vi "Get Column Config.vi"(8 "error in (no error)":errorcluster, 11 "Table Configuration Interface in":refnum<class "Table Configuration Interface.lvclass">) -> (0 "error out":errorcluster, 2 "Column Configuration":refnum<class "Column Configuration.lvclass">, 3 "Table Configuration Interface out":refnum<class "Table Configuration Interface.lvclass">)   [LabVIEW 2020, in "Table.lvlib" / "Table Configuration Interface.lvclass"]
uses:
  Table Configuration Interface.lvclass
  Column Libraries/Basic Columns/Column Configuration/Basic Column Configuration Class/Column Configuration.lvclass
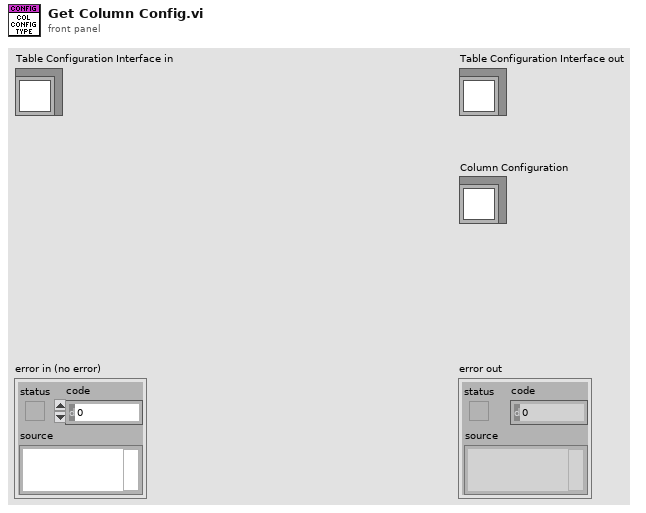
[diagram p1: front panel]
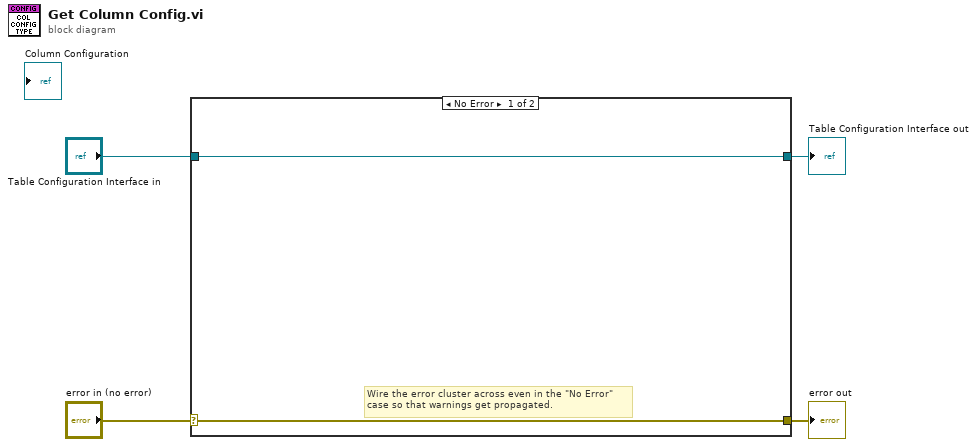
[diagram p0: block diagram]
diagram:
  n1 = case shown="No Error" "error in (no error)" {
    selector: "error in (no error)" -> [w5 w8]
    tunnel: [w5 w8] -> w3
    tunnel: [w6 w7] -> w1
    tunnel: "Table Configuration Interface in" -> [w6 w7]
    frame No Error {
      # "Wire the error cluster across even in the \"No Error\"\ncase so that warnings get propagated."
    }
    frame Error {
    }
  }
  "error out" <- w3
  "Table Configuration Interface out" <- w1
